vi "8 Bits Initialize Entry.vi"(6 "E?E1:E2 (E1)":bool=TRUE, 11 "device connection map":T1={"RS"="RS", "R/W"="RW", "E1"="E1", "E2"="E1", "DB0"="DB0", "DB1"="DB1", "DB2"="DB2", "DB3"="DB3", "DB4"="DB4", "DB5"="DB5", "DB6"="DB6", "DB7"="DB7"}) -> ()   [LabVIEW 2017, in "HD44780 FPGA.lvlib"]
uses:
  HD44780 FPGA.lvlib
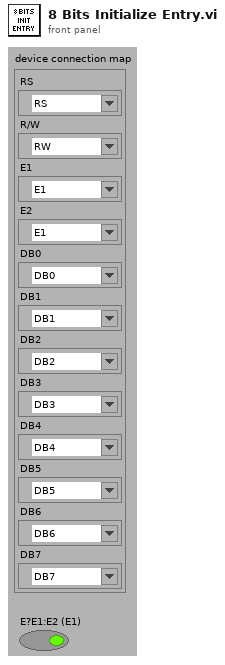
[diagram p1: front panel]
types:
  T1 = cluster{"RS":refnum<k21>, "R/W":refnum<k21>, "E1":refnum<k21>, "E2":refnum<k21>, "DB0":refnum<k21>, "DB1":refnum<k21>, "DB2":refnum<k21>, "DB3":refnum<k21>, "DB4":refnum<k21>, "DB5":refnum<k21>, "DB6":refnum<k21>, "DB7":refnum<k21>}
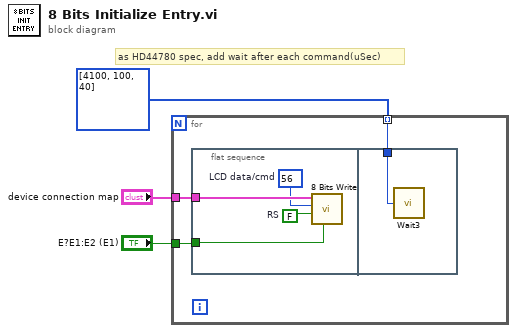
[diagram p0: block diagram]
diagram:
  # "as HD44780 spec, add wait after each command(uSec)"
  n1 = for {
    tunnel: "device connection map" -> [w6]
    tunnel: "E?E1:E2 (E1)" -> [w5]
    tunnel: u16[] [4100, 100, 40] ("initialized array") -> [w4] mode=indexing
    n2 = flat-sequence {
      tunnel: w6 -> [w9]
      tunnel: w5 -> [w8]
      tunnel: w4 -> [w11]
      frame #0 {
        w7 = u8 56  # LCD data/cmd
        w10 = FALSE  # RS
        n3 = call "8 Bits Write.vi"("E?E1:E2 (E1)"=w8, "RS"=w10, "LCD data/cmd"=w7, "device connection map"=w9) -> ()  [unwired: 8 in]
      }
      frame #1 {
        n4 = call "Wait3"("Count(uSec)"=w11) -> ()  [unwired: 1 out]
      }
    }
  }
